vi "analyzeToolingPins.vi"() -> ()   [LabVIEW 2016]
uses:
  <vilib>/Utility/file.llb/Read Delimited Spreadsheet (DBL).vi
  <vilib>/Utility/file.llb/Write Delimited Spreadsheet (DBL).vi
  <vilib>/vision/NI_Vision_Development_Module.lvlib
  <vilib>/Analysis/NI_AALPro.lvlib
panel:
  in  "write path (dialog if empty) 2":path=path "E:/XYZstage+Camera_CollectedImages/12-12-2016/pinLocations_Global-noAve.csv"
  in  "write path (dialog if empty)":path=path "E:/XYZstage+Camera_CollectedImages/12-12-2016/pinLocations_Global.csv"
  out "Pin coordinates":dbl[][](array[numeric])
  out "Parallel?":dbl[](array[numeric])=[0.7938159832357337, -0.16715013138871848, 0.17555743300974758, 1.221070473447642, 0.5717372692283367]
  out "Bottom lines":T1(array[cluster])=[{"Point1 (Pixels)"={"X"=588.0, "Y"=1498.978}, "Point2 (Pixels)"={"X"=2568.0, "Y"=1507.6019}, "Point1 (Real-World)"={"X"=1465.9109, "Y"=-3774.6116}, "Point2 (Real-World)"={"X"=8062.4556, "Y"=-3803.3218}, "Angle (Pixel)"=-0.24955172449899274, "Angle (Real-World)"=-0.24955172449899274, "Score"=87.58170183967141, "Straightness"=1.588660998181161, "Average SNR (db)"=6.1038951610625425, "Calibration Valid"=TRUE}, {"Point1 (Pixels)"={"X"=588.0, "Y"=1377.314}, "Point2 (Pixels)"={"X"=2568.0, "Y"=1425.8923}, "Point1 (Real-World)"={"X"=1465.9095, "Y"=-3369.277}, "Point2 (Real-World)"={"X"=8062.455, "Y"=-3531.099}, "Angle (Pixel)"=-1.405442823009806, "Angle (Real-World)"=-1.405442823009806, "Score"=168.62745098039215, "Straightness"=0.7396880243733882, "Average SNR (db)"=89.5444695301581, "Calibration Valid"=TRUE}, {"Point1 (Pixels)"={"X"=588.0, "Y"=1440.2833}, "Point2 (Pixels)"={"X"=2568.0, "Y"=1460.9584}, "Point1 (Real-World)"={"X"=1465.9103, "Y"=-3579.065}, "Point2 (Real-World)"={"X"=8062.455, "Y"=-3647.9248}, "Angle (Pixel)"=-0.5982586059412303, "Angle (Real-World)"=-0.5982586059412303, "Score"=104.57516090542663, "Straightness"=3.403428798938677, "Average SNR (db)"=7.278509300839606, "Calibration Valid"=TRUE}, {"Point1 (Pixels)"={"X"=588.0, "Y"=1452.9336}, "Point2 (Pixels)"={"X"=2568.0, "Y"=1451.0005}, "Point1 (Real-World)"={"X"=1465.9104, "Y"=-3621.2104}, "Point2 (Real-World)"={"X"=8062.455, "Y"=-3614.749}, "Angle (Pixel)"=0.05593523554043145, "Angle (Real-World)"=0.05593523554043145, "Score"=129.41176470588235, "Straightness"=4.674530539462709, "Average SNR (db)"=218.3133547851311, "Calibration Valid"=TRUE}, {"Point1 (Pixels)"={"X"=588.0, "Y"=1578.3824}, "Point2 (Pixels)"={"X"=2568.0, "Y"=1555.0287}, "Point1 (Real-World)"={"X"=1465.9117, "Y"=-4039.1545}, "Point2 (Real-World)"={"X"=8062.456, "Y"=-3961.3284}, "Angle (Pixel)"=0.6757647860093812, "Angle (Real-World)"=0.6757647860093812, "Score"=118.95425085927926, "Straightness"=1.2787765878925301, "Average SNR (db)"=7.118476601436699, "Calibration Valid"=TRUE}]
  out "Top lines":T1(array[cluster])=[{"Point1 (Pixels)"={"X"=672.0, "Y"=295.8632}, "Point2 (Pixels)"={"X"=2592.0, "Y"=336.42792}, "Point1 (Real-World)"={"X"=1745.7515, "Y"=233.67255}, "Point2 (Real-World)"={"X"=8142.4014, "Y"=98.54803}, "Angle (Pixel)"=-1.210334963957509, "Angle (Real-World)"=-1.210334963957509, "Score"=58.8235294117647, "Straightness"=2.4017772878485184, "Average SNR (db)"=1.1482845746428507, "Calibration Valid"=TRUE}, {"Point1 (Pixels)"={"X"=672.0, "Y"=191.64069}, "Point2 (Pixels)"={"X"=2592.0, "Y"=231.99863}, "Point1 (Real-World)"={"X"=1745.7504, "Y"=580.89905}, "Point2 (Real-World)"={"X"=8142.4004, "Y"=446.4634}, "Angle (Pixel)"=-1.2041662723693978, "Angle (Real-World)"=-1.2041662723693978, "Score"=105.88235294117646, "Straightness"=1.8960216745894505, "Average SNR (db)"=1.4967722432430375, "Calibration Valid"=TRUE}, {"Point1 (Pixels)"={"X"=672.0, "Y"=270.6548}, "Point2 (Pixels)"={"X"=2592.0, "Y"=294.97293}, "Point1 (Real-World)"={"X"=1745.7512, "Y"=317.6566}, "Point2 (Real-World)"={"X"=8142.401, "Y"=236.65897}, "Angle (Pixel)"=-0.7256522526793593, "Angle (Real-World)"=-0.7256522526793593, "Score"=32.67973731545841, "Straightness"=3.713006222858965, "Average SNR (db)"=1.613595953683743, "Calibration Valid"=TRUE}, {"Point1 (Pixels)"={"X"=672.0, "Y"=224.16507}, "Point2 (Pixels)"={"X"=2592.0, "Y"=232.6439}, "Point1 (Real-World)"={"X"=1745.7507, "Y"=472.54117}, "Point2 (Real-World)"={"X"=8142.4004, "Y"=444.31363}, "Angle (Pixel)"=-0.25301992920225524, "Angle (Real-World)"=-0.25301992920225524, "Score"=151.63399191463694, "Straightness"=0.510345166583448, "Average SNR (db)"=3.9147403634410223, "Calibration Valid"=TRUE}, {"Point1 (Pixels)"={"X"=672.0, "Y"=377.33505}, "Point2 (Pixels)"={"X"=2592.0, "Y"=324.44504}, "Point1 (Real-World)"={"X"=1745.7523, "Y"=-37.75815}, "Point2 (Real-World)"={"X"=8142.4014, "Y"=138.47005}, "Angle (Pixel)"=1.5779210691337937, "Angle (Real-World)"=1.5779210691337937, "Score"=45.751635233561196, "Straightness"=1.6378265082332055e-14, "Average SNR (db)"=7.949455824866359, "Calibration Valid"=TRUE}]
  in  "file name pattern":string="pin*_*.png"
  in  "error in (no error)":errorcluster
  in  "Calibration Image":path=path "E:/XYZstage+Camera_CollectedImages/12-12-2016/Calibration_moduleOnStave_0,2p2,0.png"
  in  "delimiter (\\t)":string=","
  out "Tooling Pin XYZ Stage Coords":dbl[][](array[numeric])
  in  "XYZ Coordinates file":path=path "E:/XYZstage+Camera_CollectedImages/12-12-2016/pinLocations_XYZ.csv"
  in  "Source images":path=path "E:/XYZstage+Camera_CollectedImages/12-12-2016"
  out "Images Array":T2[](array[plugin-control])
  # "EDGE DIAGNOSTICS"
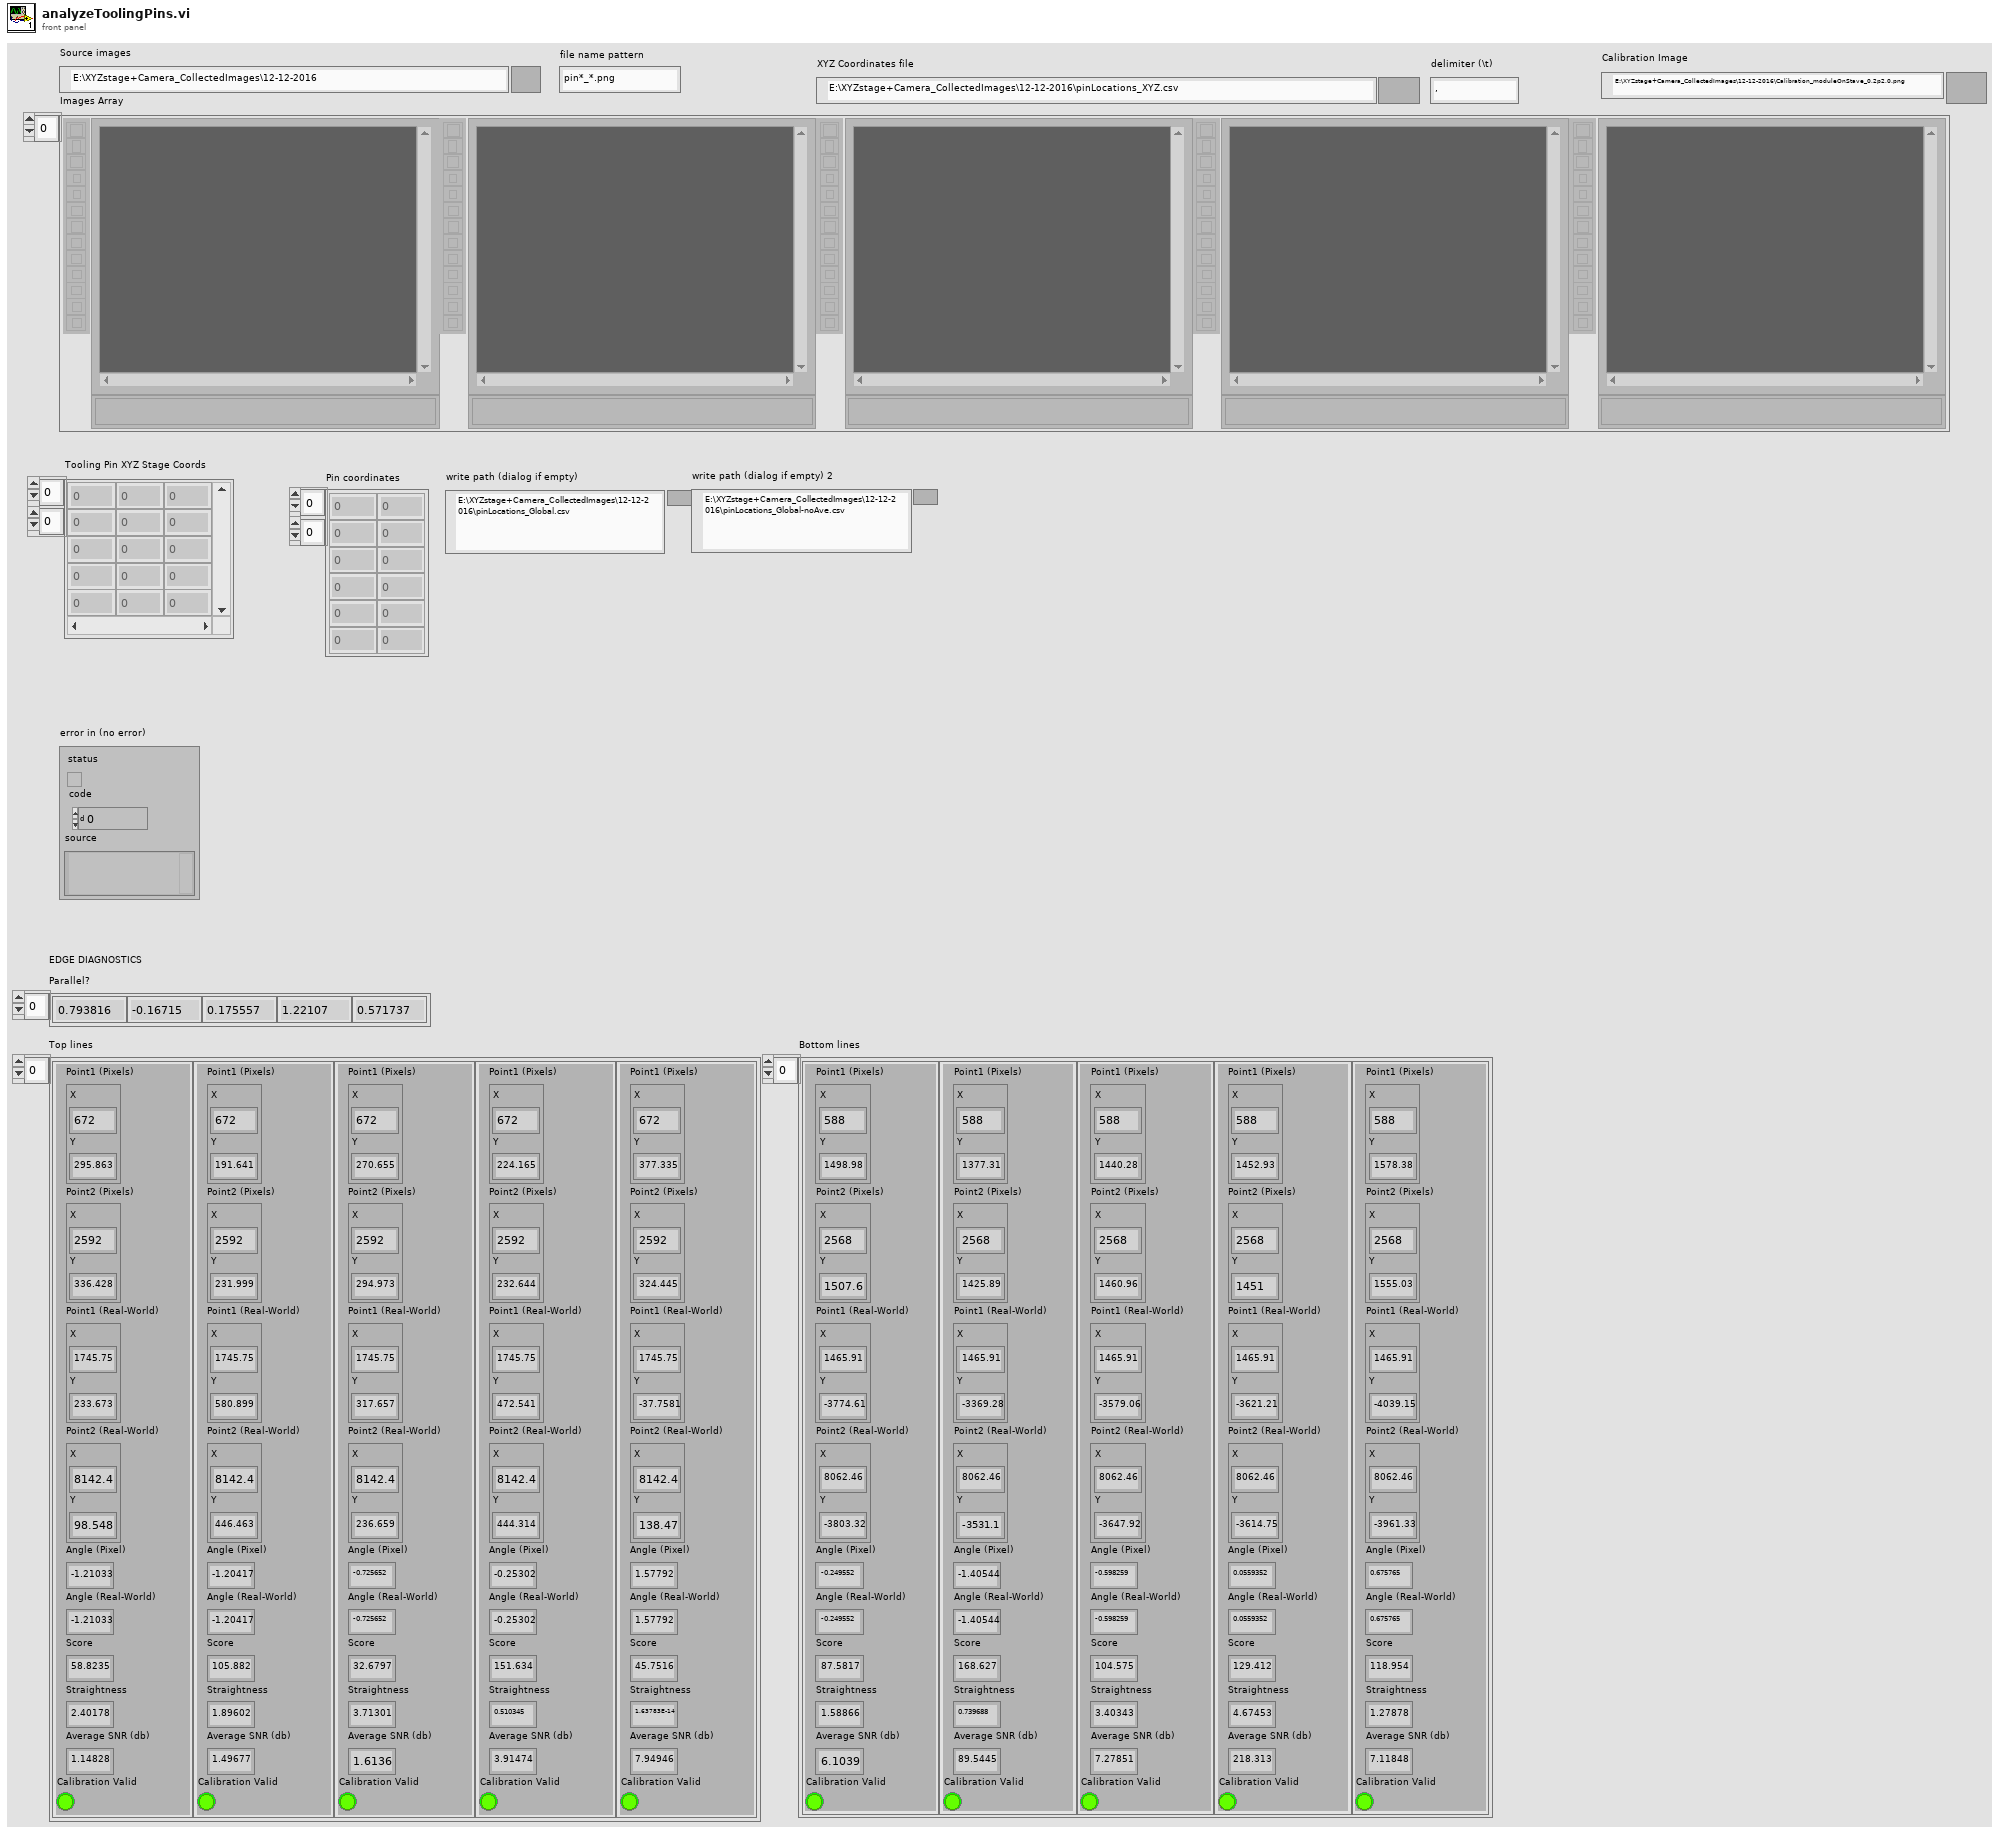
[diagram p1: front panel]
types:
  T1 = cluster{"Point1 (Pixels)":cluster{"X":sgl, "Y":sgl}, "Point2 (Pixels)":cluster{"X":sgl, "Y":sgl}, "Point1 (Real-World)":cluster{"X":sgl, "Y":sgl}, "Point2 (Real-World)":cluster{"X":sgl, "Y":sgl}, "Angle (Pixel)":dbl, "Angle (Real-World)":dbl, "Score":dbl, "Straightness":dbl, "Average SNR (db)":dbl, "Calibration Valid":bool}[]
  T2 = typedef "IMAQ Image.ctl" = refnum<image>
  T3 = cluster{"Point1 (Pixels)":cluster{"X":sgl, "Y":sgl}, "Point2 (Pixels)":cluster{"X":sgl, "Y":sgl}, "Point1 (Real-World)":cluster{"X":sgl, "Y":sgl}, "Point2 (Real-World)":cluster{"X":sgl, "Y":sgl}, "Angle (Pixel)":dbl, "Angle (Real-World)":dbl, "Score":dbl, "Straightness":dbl, "Average SNR (db)":dbl, "Calibration Valid":bool}
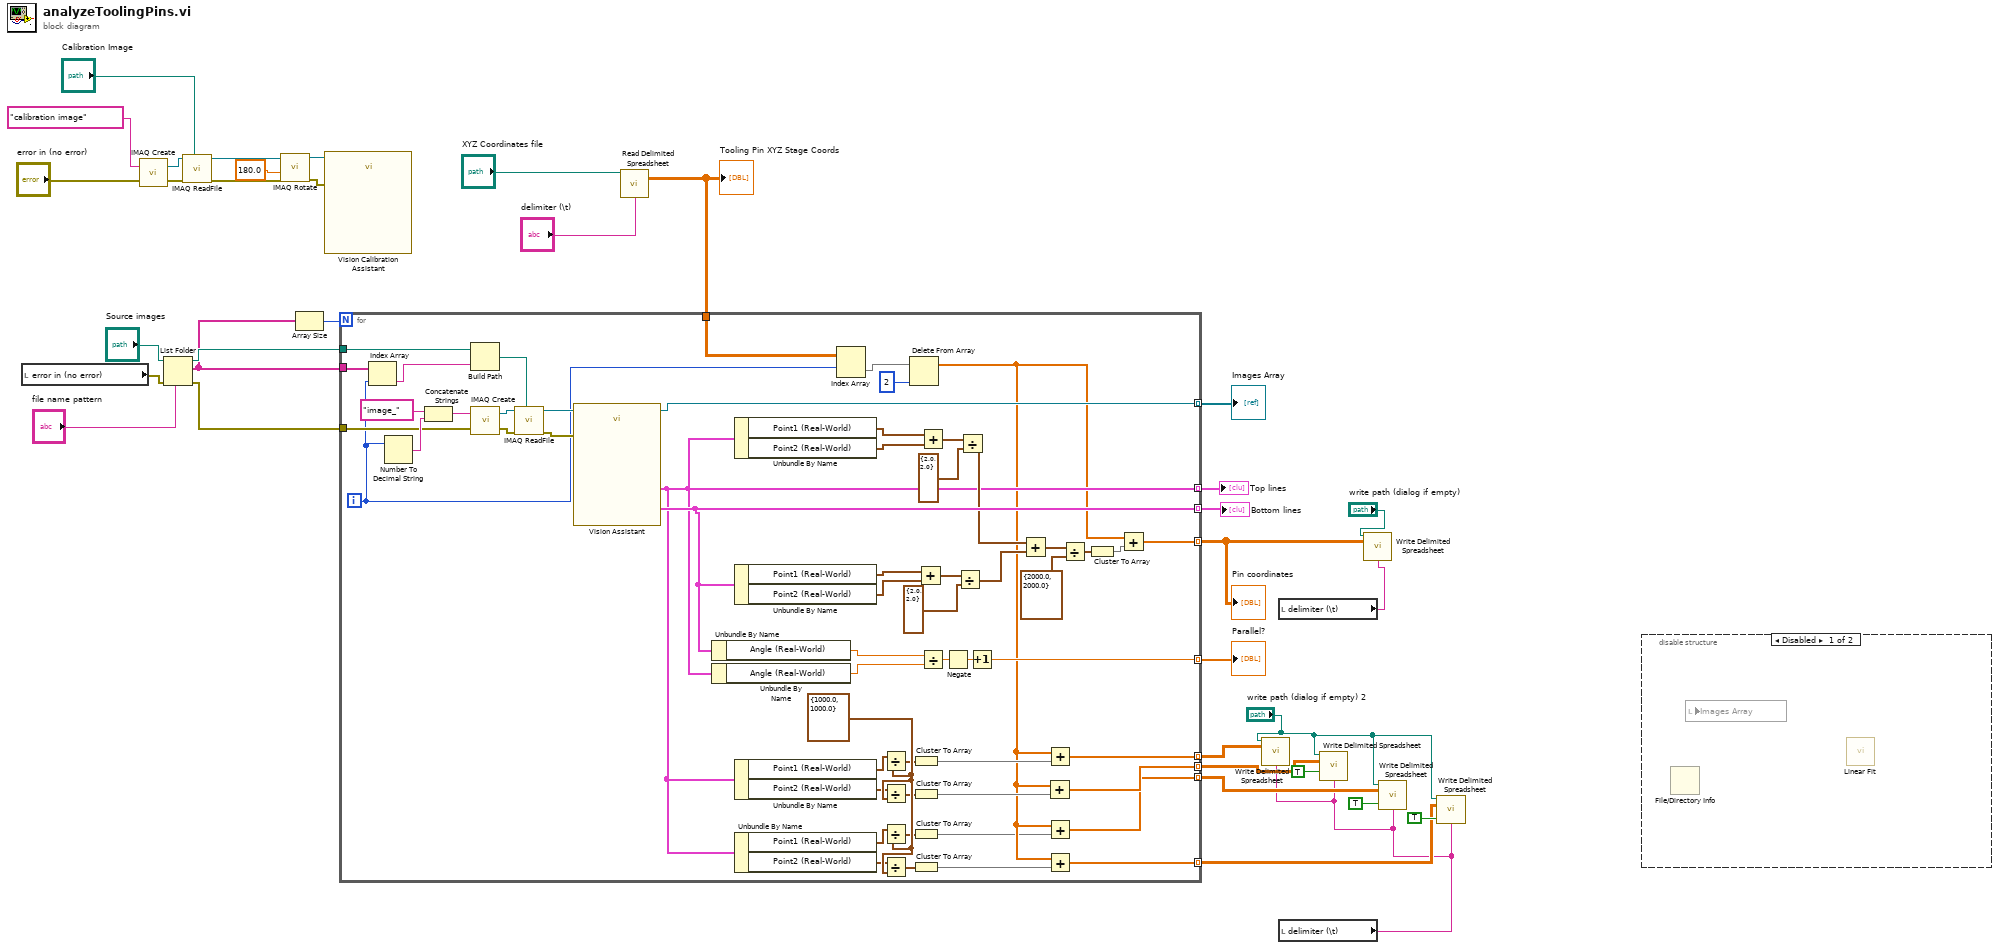
[diagram p0: block diagram]
diagram:
  n1 = local read "error in (no error)"() -> (w24:errorcluster)
  n2 = call "IMAQ Create"("Image Name"="calibration image", "error in (no error)"="error in (no error)") -> ("New Image"=w34:T2, "error out"=w35:errorcluster)  [unwired: 3 in]
  n3 = List Folder(path="Source images", pattern="file name pattern", error in=w24) -> (path out=w20:path, filenames=w19:string[], error out=w21:errorcluster)  [unwired: 1 in, 1 out]
  n4 = call "IMAQ ReadFile"("File Path"="Calibration Image", "error in (no error)"=w35, "Image"=w34) -> ("error out"=w30:errorcluster, "Image Out"=w29:T2)  [unwired: 4 in, 3 out]
  n5 = call "IMAQ Rotate"("error in (no error)"=w30, "Angle (degrees)"=sgl 180.0, "Image Src"=w29) -> ("error out"=w26:errorcluster, "Image Dst Out"=w27:T2)  [unwired: 7 in]
  n6 = Array Size(array=w19) -> (size(s)=w22:i32)
  n7 = call "Vision Calibration Assistant"("Image In"=w27, "error in"=w26) -> ()  [unwired: 24 in, 2 out]
  n8 = call-poly <vilib>:"Read Delimited Spreadsheet.vi"("file path (dialog if empty)"="XYZ Coordinates file", "delimiter (\\t)"="delimiter (\\t)") -> ("all rows"=w13:dbl[][])  [unwired: 8 in, 5 out]
  "Tooling Pin XYZ Stage Coords" <- w13
  n9 = for {
    N: w22 -> [_]
    tunnel: w21 -> [w90]
    tunnel: w20 -> [w86]
    tunnel: w19 -> [w85]
    tunnel: [w63] -> w18 mode=indexing
    tunnel: [w55] -> w17 mode=indexing
    tunnel: [w76] -> w16 mode=indexing
    tunnel: [w77] -> w15 mode=indexing
    tunnel: w13 -> [w62]
    tunnel: [w56] -> w12 mode=indexing
    tunnel: [w40] -> w9 mode=indexing
    tunnel: [w39] -> w8 mode=indexing
    tunnel: [w38] -> w4 mode=indexing
    tunnel: [w37] -> w3 mode=indexing
    i -> [w61]
    w53 = cluster{"X":sgl, "Y":sgl} {"X"=1000.0, "Y"=1000.0} ("y")
    n10 = Index Array(array=w85, index=w61) -> (element=w84:string)
    n11 = Number To Decimal String(number=w61) -> (decimal integer string=w92:string)  [unwired: 1 in]
    n12 = Concatenate Strings("image_" ("Image Name"), w92) -> (w91:string)
    n13 = Build Path(base path=w86, name or relative path=w84) -> (appended path=w87:path)
    n14 = call "IMAQ Create"("Image Name"=w91, "error in (no error)"=w90) -> ("New Image"=w88:T2, "error out"=w89:errorcluster)  [unwired: 3 in]
    n15 = call "IMAQ ReadFile"("File Path"=w87, "error in (no error)"=w89, "Image"=w88) -> ("error out"=w82:errorcluster, "Image Out"=w83:T2)  [unwired: 4 in, 3 out]
    n16 = call "Vision Assistant"("Image In"=w83, "error in"=w82) -> ("Image Out"=w63:T2, "Straight Edge (Find top straight edge)"=w55:T3, "Straight Edge (Find bottom straight edge)"=w76:T3)  [unwired: 22 in, 1 out]
    n17 = Unbundle By Name(w76) -> ("Angle (Real-World)"=w81:dbl)
    n18 = Unbundle By Name(w55) -> ("Angle (Real-World)"=w80:dbl)
    n19 = Unbundle By Name(w55) -> ("Point1 (Real-World)"=w75:cluster{"X":sgl, "Y":sgl}, "Point2 (Real-World)"=w74:cluster{"X":sgl, "Y":sgl})
    n20 = Unbundle By Name(w76) -> ("Point1 (Real-World)"=w70:cluster{"X":sgl, "Y":sgl}, "Point2 (Real-World)"=w69:cluster{"X":sgl, "Y":sgl})
    n21 = Unbundle By Name(w55) -> ("Point1 (Real-World)"=w54:cluster{"X":sgl, "Y":sgl}, "Point2 (Real-World)"=w50:cluster{"X":sgl, "Y":sgl})
    n22 = Unbundle By Name(w55) -> ("Point1 (Real-World)"=w52:cluster{"X":sgl, "Y":sgl}, "Point2 (Real-World)"=w51:cluster{"X":sgl, "Y":sgl})
    n23 = Index Array(array=w62, index (row)=w61) -> (element=w60:dbl[])  [unwired: 1 in]
    n24 = Divide(x=w54, y=w53) -> (x/y=w46:cluster{"X":sgl, "Y":sgl})
    n25 = Divide(x=w50, y=w53) -> (x/y=w47:cluster{"X":sgl, "Y":sgl})
    n26 = Divide(x=w52, y=w53) -> (x/y=w48:cluster{"X":sgl, "Y":sgl})
    n27 = Divide(x=w51, y=w53) -> (x/y=w49:cluster{"X":sgl, "Y":sgl})
    n28 = Delete From Array(array=w60, index=2) -> (array with subset deleted=w43:dbl[])  [unwired: 1 in, 1 out]
    n29 = Cluster To Array(cluster=w46) -> (array=w45:sgl[])
    n30 = Cluster To Array(cluster=w47) -> (array=w44:sgl[])
    n31 = Cluster To Array(cluster=w48) -> (array=w42:sgl[])
    n32 = Cluster To Array(cluster=w49) -> (array=w41:sgl[])
    n33 = Add(x=w70, y=w69) -> (x+y=w71:cluster{"X":sgl, "Y":sgl})
    n34 = Add(x=w75, y=w74) -> (x+y=w73:cluster{"X":sgl, "Y":sgl})
    n35 = Divide(x=w81, y=w80) -> (x/y=w79:dbl)
    n36 = Negate(x=w79) -> (-x=w78:dbl)
    n37 = Divide(x=w71, y=cluster{"X":sgl, "Y":sgl} {"X"=2.0, "Y"=2.0}) -> (x/y=w66:cluster{"X":sgl, "Y":sgl})
    n38 = Divide(x=w73, y=cluster{"X":sgl, "Y":sgl} {"X"=2.0, "Y"=2.0}) -> (x/y=w67:cluster{"X":sgl, "Y":sgl})
    n39 = Increment(x=w78) -> (x+1=w77:dbl)
    n40 = Add(x=w67, y=w66) -> (x+y=w68:cluster{"X":sgl, "Y":sgl})
    n41 = Add(x=w43, y=w44) -> (x+y=w39:dbl[])
    n42 = Add(x=w43, y=w45) -> (x+y=w40:dbl[])
    n43 = Add(x=w43, y=w42) -> (x+y=w38:dbl[])
    n44 = Add(x=w43, y=w41) -> (x+y=w37:dbl[])
    n45 = Divide(x=w68, y=cluster{"X":sgl, "Y":sgl} {"X"=2000.0, "Y"=2000.0}) -> (x/y=w58:cluster{"X":sgl, "Y":sgl})
    n46 = Cluster To Array(cluster=w58) -> (array=w57:sgl[])
    n47 = Add(x=w43, y=w57) -> (x+y=w56:dbl[])
  }
  "Images Array" <- w18
  "Top lines" <- w17
  "Bottom lines" <- w16
  "Parallel?" <- w15
  "Pin coordinates" <- w12
  n48 = local read "delimiter (\\t)"() -> (w11:string)
  n49 = local read "delimiter (\\t)"() -> (w2:string)
  n50 = call-poly <vilib>:"Write Delimited Spreadsheet.vi"("file path (dialog if empty)"="write path (dialog if empty) 2", "2D data"=w9, "delimiter (\\t)"=w2) -> ()  [unwired: 11 in, 2 out]
  n51 = call-poly <vilib>:"Write Delimited Spreadsheet.vi"("file path (dialog if empty)"="write path (dialog if empty) 2", "2D data"=w8, "append to file? (new file:F)"=TRUE, "delimiter (\\t)"=w2) -> ()  [unwired: 10 in, 2 out]
  n52 = call-poly <vilib>:"Write Delimited Spreadsheet.vi"("file path (dialog if empty)"="write path (dialog if empty)", "2D data"=w12, "delimiter (\\t)"=w11) -> ()  [unwired: 11 in, 2 out]
  n53 = call-poly <vilib>:"Write Delimited Spreadsheet.vi"("file path (dialog if empty)"="write path (dialog if empty) 2", "2D data"=w4, "append to file? (new file:F)"=TRUE, "delimiter (\\t)"=w2) -> ()  [unwired: 10 in, 2 out]
  n54 = call-poly <vilib>:"Write Delimited Spreadsheet.vi"("file path (dialog if empty)"="write path (dialog if empty) 2", "2D data"=w3, "append to file? (new file:F)"=TRUE, "delimiter (\\t)"=w2) -> ()  [unwired: 10 in, 2 out]
  n55 = disable-structure shown="Disabled" {
    frame Disabled {
      n56 = File/Directory Info() -> ()  [unwired: 2 in, 7 out]
      n57 = local read "Images Array"() -> ()  [unwired: 1 in]
      n58 = call <vilib>:"Linear Fit.vi"() -> ()  [unwired: 11 in, 5 out]
    }
    frame Enabled {
    }
  }
